vi "MOV_Query_old.vi"(0 "System no.":i32=1 min=1 max=4 step=1, 5 "error in":errorcluster, 12 "Stop refnum":refnum<vi>) -> (14 "Moving?":bool, 19 "error out":errorcluster)   [LabVIEW 2020]
doc: "Sends MOV? and waits for response of 0 (not moving). In case of no answer, VI stops after 60 s.VI also stops if Local stop or Stop refnum is TRUE. When using as a sub-VI, use Stop refnum to stop VI from caller.\n\nF-206, M-8X0: Only for GCS syntax version = GCS 1.0 (check with CSV?.vi. If CSV?.vi is not supported, syntax version is GCS 1.0)."
panel:
  in  "Local stop":bool
  # "Old command declaration! Sends MOV? and waits for \nresponse of 0 (not moving). In case of no answer, vi \nstops after 60s. VI also stops if Local stop or Stop \nrefnum is TRUE."
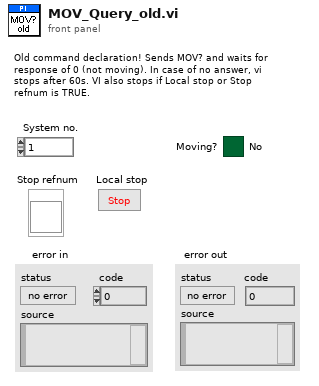
[diagram p1: front panel]
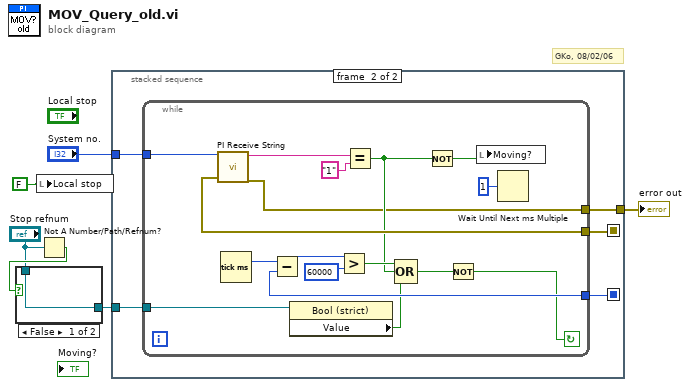
[diagram p0: block diagram]
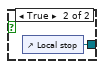
[diagram p2: hidden frame]
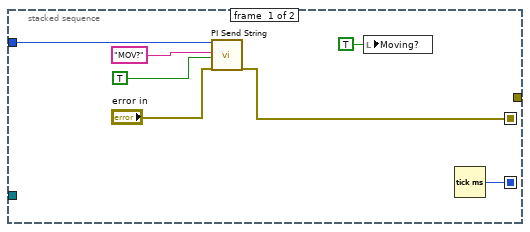
[diagram p3: hidden frame]
diagram:
  # "GKo, 08/02/06"
  n1 = local write "Local stop"(FALSE ("Local stop")) -> ()
  n2 = Not A Number/Path/Refnum?(number/path/refnum="Stop refnum") -> (NaN/Path/Refnum?=w4:bool)
  n3 = case shown="False" w4 {
    tunnel: "Stop refnum" -> [w7 _]
    tunnel: [w7 w8] -> w1
    frame False {
    }
    frame True {
      n4 = control-ref of="Local stop"() -> (w8:refnum<vi>)
    }
  }
  n5 = stacked-sequence {
    seq-local: [w13 _] -> [_ w20]
    seq-local: [w9 _] -> [_ w18]
    tunnel: "System no." -> [w10 w19]
    tunnel: [_ w17] -> w5
    tunnel: w1 -> [_ w16]
    frame #0 {
      n6 = call "PI Send String.vi"("System no."=w10, "String to send"="MOV?", "Attach termination char.?"=TRUE ("Attach Linefeed?"), "error in"="error in") -> ("error out"=w13:errorcluster)  [unwired: 15 out]
      n7 = local write "Moving?"(TRUE ("Moving?")) -> ()
      n8 = Tick Count (ms)() -> (millisecond timer value=w9:u32)
    }
    frame #1 {
      n9 = while {
        tunnel: w16 -> [w22]
        tunnel: [w24] -> w17
        tunnel: w18 -> [w32]
        tunnel: w19 -> [w34]
        tunnel: w20 -> [w37]
        stop <- w26 continue-if-true
        n10 = call "PI Receive String.vi"("System no."=w34, "error in"=w37) -> ("String read"=w36:string, "error out"=w24:errorcluster)  [unwired: 1 in, 15 out]
        n11 = Tick Count (ms)() -> (millisecond timer value=w33:u32)
        n12 = Subtract(x=w33, y=w32) -> (x-y=w31:u32)
        n13 = property class="Bool (strict)"(reference=w22) -> ("Value"=w23:bool)  [unwired: 1 in, 2 out]
        n14 = Greater?(x=w31, y=u32 60000) -> (0:w29:bool)
        n15 = Equal?(x=w36, y="1") -> (x = y?=w28:bool)
        n16 = Compound Arithmetic op=OR(w29, w28, w23) -> (w27:bool)
        n17 = Not(x=w28) -> (.not. x?=w35:bool)
        n18 = Not(x=w27) -> (.not. x?=w26:bool)
        n19 = local write "Moving?"(w35) -> ()
        n20 = Wait Until Next ms Multiple(millisecond multiple=u32 1) -> ()  [unwired: 1 out]
      }
    }
  }
  "error out" <- w5
